vi "provide_OME_data.vi"(6 "image ID":string, 8 "error in (no error)":errorcluster, 9 "structuredAttribute string in":string, 10 "OME element in":refnum<class "XMLElement.lvclass">, 11 "LightSourceDL090909Filament in":refnum<class "LightSourceDL090909Filament.lvclass">) -> (0 "error out":errorcluster, 1 "structuredAttribute string out":string, 2 "OME element out":refnum<class "XMLElement.lvclass">, 3 "LightSourceDL090909Filament out":refnum<class "LightSourceDL090909Filament.lvclass">)   [LabVIEW 2010, in "LightSourceDL090909Filament.lvclass"]
uses:
  LightSourceDL090909Filament.lvclass
  common/classes/XMLElement/XMLElement/XMLElement.lvclass
  GenericLightSource/GenericLightSource/GenericLightSource.lvclass
  LightSourceDL090909Filament.lvclass/LightSourceDL090909Filament.ctl
  Instrument/GenericInstrument/GenericInstrument/GenericInstrument.lvclass
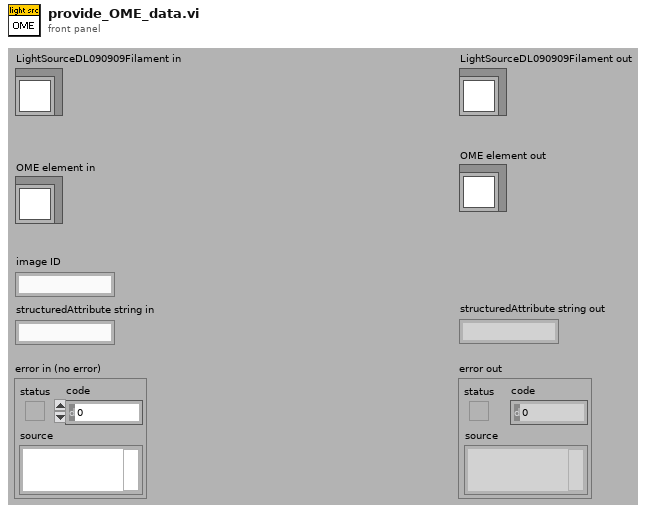
[diagram p1: front panel]
types:
  T1 = typedef "LightSourceDL090909Filament.lvclass/type_enum.ctl" = enum16{"Incandescent", "Halogen", "Unknown"}
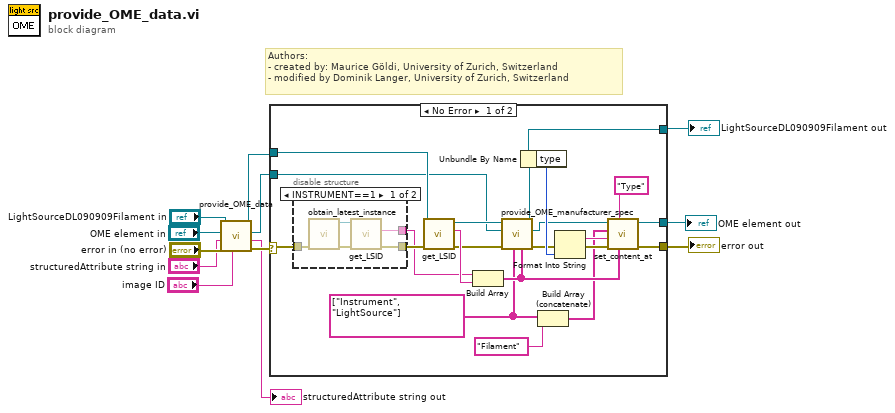
[diagram p0: block diagram]
diagram:
  # "Authors: \n- created by: Maurice Göldi, University of Zurich, Switzerland\n- modified by Dominik Langer, University of Zurich, Switzerland"
  n1 = call-parent "provide_OME_data.vi"("image ID"="image ID", "error in (no error)"="error in (no error)", "structuredAttribute string in"="structuredAttribute string in", "OME element in"="OME element in", "GenericPlugin in"="LightSourceDL090909Filament in") -> ("error out"=w8:errorcluster, "structuredAttribute string out"=→"structuredAttribute string out":string, "OME element out"=w10:refnum<class "XMLElement.lvclass">, "GenericPlugin out"=w9:refnum<class "LightSourceDL090909Filament.lvclass">)  [unwired: 3 in]
  n2 = case shown="No Error" w8 {
    selector: w8 -> [w26 w40]
    tunnel: w10 -> [w17 w41]
    tunnel: w9 -> [w25 w42]
    tunnel: [w19 w42] -> w6
    tunnel: [w30 w40] -> w7
    tunnel: [w29 w41] -> w4
    frame No Error {
      w14 = string[] ["Instrument", "LightSource"]
      n3 = disable-structure shown="INSTRUMENT==1" {
        disable-tunnel: w26 -> [w36 w39]
        disable-tunnel: [w35 w39] -> w28
        disable-tunnel: [w34 _] -> w27
        frame condition #0 {
          n4 = call "obtain_latest_instance.vi"("error in (no error)"=w36) -> ("error out"=w37:errorcluster, "microscope"=w38:refnum<class "GenericInstrument.lvclass">)  [unwired: 9 in]
          n5 = call-dynamic "get_LSID.vi"("error in (no error)"=w37, "GenericPlugin in"=w38) -> ("error out"=w35:errorcluster, "LSID (string)"=w34:string)  [unwired: 6 in, 2 out]
        }
        frame condition #1 (active) {
        }
      }
      n6 = call-dynamic "get_LSID.vi"("error in (no error)"=w28, "GenericPlugin in"=w25) -> ("error out"=w22:errorcluster, "LSID (string)"=w33:string, "GenericPlugin out"=w20:refnum<class "LightSourceDL090909Filament.lvclass">)  [unwired: 6 in, 1 out]
      n7 = Build Array(w27, w33) -> (w18:string[])
      n8 = call-dynamic "provide_OME_manufacturer_spec.vi"("id chain"=w18, "key chain"=w14, "error in (no error)"=w22, "XMLElement in"=w17, "GenericPlugin in"=w20) -> ("error out"=w21:errorcluster, "XMLElement out"=w16:refnum<class "XMLElement.lvclass">, "GenericPlugin out"=w19:refnum<class "LightSourceDL090909Filament.lvclass">)  [unwired: 4 in]
      n9 = Unbundle By Name(w19) -> ("type"=w32:T1)
      n10 = Build Array (concatenate)(w14, "Filament") -> (w13:string[])
      n11 = Format Into String(error in=w21, w32) -> (resulting string=w24:string, error out=w31:errorcluster)  [unwired: 2 in]
      n12 = call "set_content_at.vi"("id chain"=w18, "attribute name"="Type" ("String"), "error in (no error)"=w31, "content"=w24, "key chain"=w13, "Element in"=w16) -> ("error out"=w30:errorcluster, "Element out"=w29:refnum<class "XMLElement.lvclass">)  [unwired: 4 in]
    }
    frame Error {
    }
  }
  "error out" <- w7
  "LightSourceDL090909Filament out" <- w6
  "OME element out" <- w4
